vi "Hatch Panel Intake.vi"   [LabVIEW 2018]
uses:
  <vilib>/Rock Robotics/WPI/Solenoid/WPI_SolenoidChannel.ctl
  <vilib>/Rock Robotics/WPI/Solenoid/WPI_SolenoidValue.ctl
  Hatch Panel Intake Global.vi
  <vilib>/Rock Robotics/WPI/Solenoid/WPI_SolenoidOpenSingle.vi
  Controllers/Manipulator Controlller/Manipulator Controller Global.vi
  <vilib>/Rock Robotics/WPI/Solenoid/WPI_SolenoidSetEnum.vi
  Cargo Intake/Cargo Intake Global.vi
  Times/Times Global.vi
types:
  T1 = typedef "WPI_SolenoidChannel.ctl" = enum8{"Solenoid 0", "Solenoid 1", "Solenoid 2", "Solenoid 3", "Solenoid 4", "Solenoid 5", "Solenoid 6", "Solenoid 7", "Invalid"}
  T2 = enum16{"Full Manual Control", "Manual Control", "Autonomous Control", "Fully Autonomous Control"}
  T3 = typedef "WPI_SolenoidValue.ctl" = enum16{"Off", "On", "Forward", "Reverse"}
  T4 = typedef "WPI_SolenoidDevRef.ctl" = cluster{"DevStatus":errorcluster, "Pneumatics Control Module":u8, "Forward Solenoid Channel":T1, "Reverse Solenoid Channel":T1}
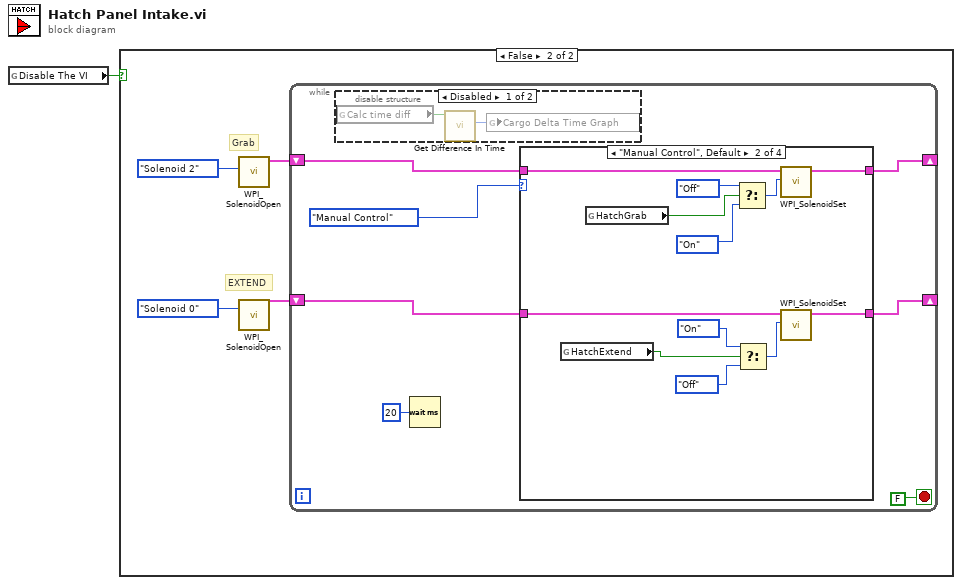
[diagram p0: block diagram]
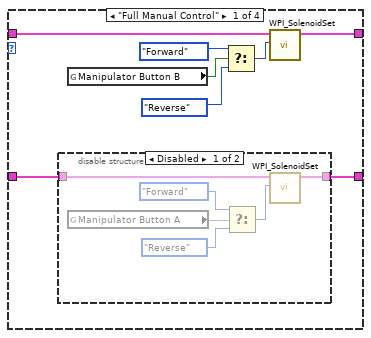
[diagram p4: hidden frame]
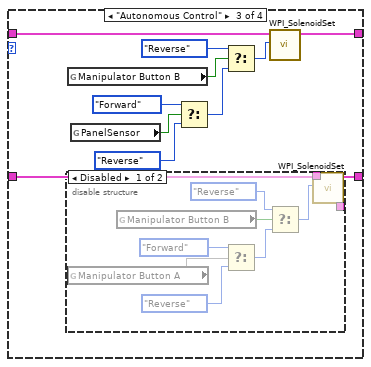
[diagram p6: hidden frame]
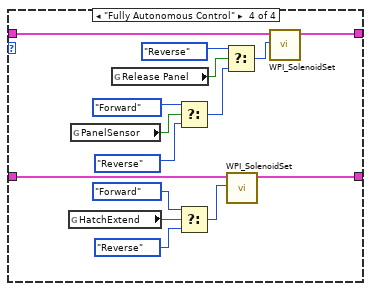
[diagram p8: hidden frame]
diagram:
  n1 = global read "Hatch Panel Intake Global.vi" "Disable The VI"() -> (w1:bool)
  n2 = case shown="False" w1 {
    frame True {
    }
    frame False {
      # "EXTEND"
      # "Grab"
      n3 = call-poly <vilib>:"WPI_SolenoidOpen.vi"("Solenoid Channel"=WPI_SolenoidChannel."Solenoid 2" ("Forward Solenoid Channel")) -> ("SolenoidDevRef"=w2:T4)  [unwired: 9 in, 1 out]
      n4 = call-poly <vilib>:"WPI_SolenoidOpen.vi"("Solenoid Channel"=WPI_SolenoidChannel."Solenoid 0" ("Forward Solenoid Channel")) -> ("SolenoidDevRef"=w5:T4)  [unwired: 9 in, 1 out]
      n5 = while {
        shift-right: [w8] -> _
        shift-left: w2 -> [w9]
        shift-right: [w7] -> _
        shift-left: w5 -> [w10]
        stop <- FALSE stop-if-true
        n6 = disable-structure shown="Disabled" {
          frame Disabled {
            n7 = global read "Cargo Intake Global.vi" "Calc time diff"() -> (w14:bool)
            n8 = call "Get Difference In Time.vi"("Calculate Time Difference"=w14) -> ("Delta Time over Time"=w13:u32)  [unwired: 9 in, 1 out]
            n9 = global write "Times Global.vi" "Cargo Delta Time Graph"(w13) -> ()
          }
          frame Enabled {
          }
        }
        n10 = Wait (ms)(milliseconds to wait=u32 20) -> ()  [unwired: 1 out]
        n11 = case shown="\"Manual Control\", Default" T2."Manual Control" ("Mode") {
          tunnel: w10 -> [w18 w35 w49 w73]
          tunnel: w9 -> [w17 w34 w51 w74]
          tunnel: [w15 w32 w50 w75] -> w8
          tunnel: [w16 w33 w48 w72] -> w7
          frame "Full Manual Control" {
            n12 = disable-structure shown="Disabled" {
              disable-tunnel: w18 -> [w24 _]
              disable-tunnel: [w23 _] -> w16
              frame Disabled {
                n13 = global read "Manipulator Controller Global.vi" "Manipulator Button A"() -> (w25)
                n14 = Select(t=WPI_SolenoidValue."Forward" ("Value"), s=w25, f=WPI_SolenoidValue."Reverse" ("Value")) -> (s? t:f=w26:T3)
                n15 = call-poly <vilib>:"WPI_SolenoidSet.vi"("Value"=w26, "SolenoidDevRef"=w24) -> ("SolenoidDevRef"=w23:T4)  [unwired: 8 in, 1 out]
              }
              frame Enabled {
              }
            }
            n16 = global read "Manipulator Controller Global.vi" "Manipulator Button B"() -> (w20:bool)
            n17 = Select(t=WPI_SolenoidValue."Forward" ("Value"), s=w20, f=WPI_SolenoidValue."Reverse" ("Value")) -> (s? t:f=w19:T3)
            n18 = call-poly <vilib>:"WPI_SolenoidSet.vi"("Value"=w19, "SolenoidDevRef"=w17) -> ("SolenoidDevRef"=w15:T4)  [unwired: 8 in, 1 out]
          }
          frame "Manual Control", Default {
            n19 = global read "Hatch Panel Intake Global.vi" "HatchExtend"() -> (w29:bool)
            n20 = global read "Hatch Panel Intake Global.vi" "HatchGrab"() -> (w30:bool)
            n21 = Select(t=WPI_SolenoidValue."Off" ("Value"), s=w30, f=WPI_SolenoidValue."On" ("Value")) -> (s? t:f=w36:T3)
            n22 = Select(t=WPI_SolenoidValue."On" ("Value"), s=w29, f=WPI_SolenoidValue."Off" ("Value")) -> (s? t:f=w39:T3)
            n23 = call-poly <vilib>:"WPI_SolenoidSet.vi"("Value"=w36, "SolenoidDevRef"=w34) -> ("SolenoidDevRef"=w32:T4)  [unwired: 8 in, 1 out]
            n24 = call-poly <vilib>:"WPI_SolenoidSet.vi"("Value"=w39, "SolenoidDevRef"=w35) -> ("SolenoidDevRef"=w33:T4)  [unwired: 8 in, 1 out]
          }
          frame "Autonomous Control" {
            n25 = disable-structure shown="Disabled" {
              disable-tunnel: w49 -> [w60 _]
              disable-tunnel: [w59 _] -> w48
              frame Disabled {
                n26 = global read "Manipulator Controller Global.vi" "Manipulator Button A"() -> (w53)
                n27 = global read "Manipulator Controller Global.vi" "Manipulator Button B"() -> (w57:bool)
                n28 = Select(t=WPI_SolenoidValue."Forward" ("Value"), s=w53, f=WPI_SolenoidValue."Reverse" ("Value")) -> (s? t:f=w54:T3)
                n29 = Select(t=WPI_SolenoidValue."Reverse" ("Value"), s=w57, f=w54) -> (s? t:f=w52:T3)
                n30 = call-poly <vilib>:"WPI_SolenoidSet.vi"("Value"=w52, "SolenoidDevRef"=w60) -> ("SolenoidDevRef"=w59:T4)  [unwired: 8 in, 1 out]
              }
              frame Enabled {
              }
            }
            n31 = global read "Manipulator Controller Global.vi" "Manipulator Button B"() -> (w47:bool)
            n32 = global read "Hatch Panel Intake Global.vi" "PanelSensor"() -> (w46:bool)
            n33 = Select(t=WPI_SolenoidValue."Forward" ("Value"), s=w46, f=WPI_SolenoidValue."Reverse" ("Value")) -> (s? t:f=w45:T3)
            n34 = Select(t=WPI_SolenoidValue."Reverse", s=w47, f=w45) -> (s? t:f=w41:T3)
            n35 = call-poly <vilib>:"WPI_SolenoidSet.vi"("Value"=w41, "SolenoidDevRef"=w51) -> ("SolenoidDevRef"=w50:T4)  [unwired: 8 in, 1 out]
          }
          frame "Fully Autonomous Control" {
            n36 = global read "Hatch Panel Intake Global.vi" "HatchExtend"() -> (w62:bool)
            n37 = global read "Hatch Panel Intake Global.vi" "PanelSensor"() -> (w69:bool)
            n38 = global read "Hatch Panel Intake Global.vi" "Release Panel"() -> (w66:bool)
            n39 = Select(t=WPI_SolenoidValue."Forward" ("Value"), s=w69, f=WPI_SolenoidValue."Reverse" ("Value")) -> (s? t:f=w68:T3)
            n40 = Select(t=WPI_SolenoidValue."Forward" ("Value"), s=w62, f=WPI_SolenoidValue."Reverse" ("Value")) -> (s? t:f=w63:T3)
            n41 = Select(t=WPI_SolenoidValue."Reverse", s=w66, f=w68) -> (s? t:f=w67:T3)
            n42 = call-poly <vilib>:"WPI_SolenoidSet.vi"("Value"=w63, "SolenoidDevRef"=w73) -> ("SolenoidDevRef"=w72:T4)  [unwired: 8 in, 1 out]
            n43 = call-poly <vilib>:"WPI_SolenoidSet.vi"("Value"=w67, "SolenoidDevRef"=w74) -> ("SolenoidDevRef"=w75:T4)  [unwired: 8 in, 1 out]
          }
        }
      }
    }
  }
